vi "TestRole_Init.vi"(0 "object in":refnum<class "TestRole.lvclass">, 5 "error in (no error)":errorcluster) -> (14 "object out":refnum<class "TestRole.lvclass">, 19 "error out":errorcluster)   [LabVIEW 2023, in "TestRole.lvclass"]
uses:
  TestRole.lvclass
  TestRole.lvclass/TestRole.ctl
  Role_class/Role.lvclass/Role.ctl
  Role_class/Read Tacticbook.vi
  Tacticbook_class/Read TestTactic.vi
  Tacticbook_class/Tacticbook.lvclass
  TestTactic_class/TestTactic.lvclass
  Role_class/Role.lvclass
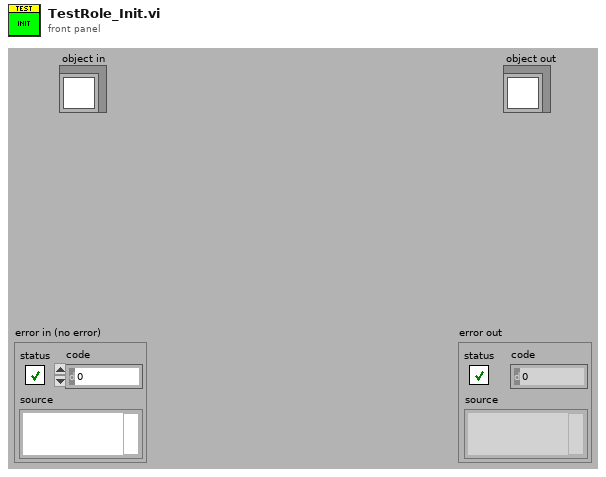
[diagram p1: front panel]
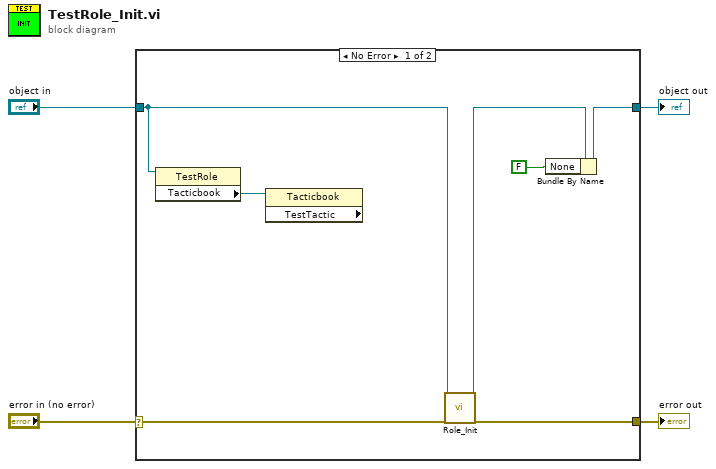
[diagram p0: block diagram]
diagram:
  n1 = case shown="No Error" "error in (no error)" {
    selector: "error in (no error)" -> [w9 w12]
    tunnel: [w11 w13] -> w4
    tunnel: "object in" -> [w6 w13]
    tunnel: [w8 w12] -> w1
    frame No Error {
      n2 = property class="TestRole"(reference=w6) -> ("Tacticbook"=w5:refnum<class "Tacticbook.lvclass">)  [unwired: 1 in, 2 out]
      n3 = property class="Tacticbook" props=["TestTactic"](reference=w5) -> ()  [unwired: 1 in, 3 out]
      n4 = call "Role_Init.vi"("object in"=w6, "error in (no error)"=w9) -> ("object out"=w7:refnum<class "TestRole.lvclass">, "error out"=w8:errorcluster)  [unwired: 16 in]
      n5 = Bundle By Name(cluster=w7, "None"=FALSE) -> (w11:refnum<class "TestRole.lvclass">)
    }
    frame Error {
    }
  }
  "object out" <- w4
  "error out" <- w1
